vi "WriteOrDestroyStream.vi"(6 "LoopCount":i32, 7 "Clust":T2, 8 "error in (no error)":errorcluster, 9 "Connected":bool, 10 "DataToSend":cluster{"QElmnt":T1, "Data":variant}={"QElmnt"=enum."RTMain_Config", "Data"=variant}, 11 "ref":refnum<k21>) -> (0 "error out":errorcluster, 3 "ref":refnum<k21>)   [LabVIEW 2018]
uses:
  Controls/StreamLoopClust.ctl
  RT/Queue/RTMainQueueElements.ctl
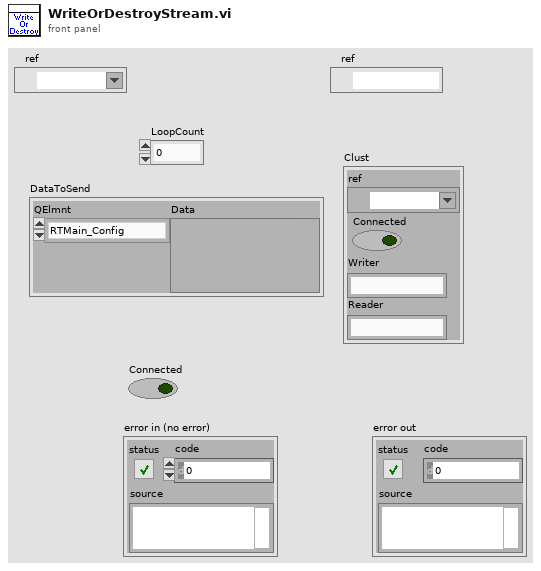
[diagram p1: front panel]
types:
  T1 = typedef "RTMainQueueElements.ctl" = enum16{"RTMain_InitQ", "RTMain_InitSW", "RTMain_InitCtrls", "RTMain_ReInitHW", "RTMain_FromStream", "RTMain_StrtHWLp", "RTMain_UpdtHWClstr", "RTMain_Start", "RTMain_Stop", "RTMain_Error", "RTMain_Config", "RTMain_Exit"}
  T2 = typedef "StreamLoopClust.ctl" = cluster{"ref":refnum<k21>, "Connected":bool, "Writer":string, "Reader":string}
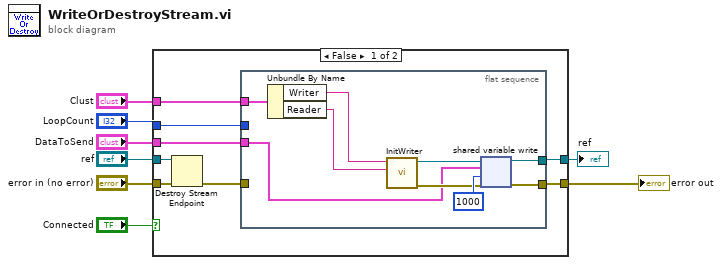
[diagram p0: block diagram]
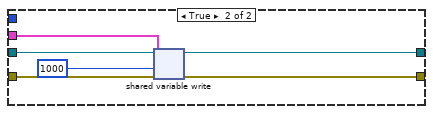
[diagram p2: hidden frame]
diagram:
  n1 = case shown="False" "Connected" {
    tunnel: [w13 w29] -> w1
    tunnel: [w14 w28] -> w6
    tunnel: "DataToSend" -> [w9 w31]
    tunnel: "ref" -> [w15 w26]
    tunnel: "error in (no error)" -> [w16 w30]
    tunnel: "Clust" -> [w12 _]
    tunnel: "LoopCount" -> [w11 _]
    frame False {
      n2 = Destroy Stream Endpoint(8:w16, 11:w15) -> (0:w10:errorcluster)
      n3 = flat-sequence {
        tunnel: [w24] -> w14
        tunnel: [w23] -> w13
        tunnel: w12 -> [w20]
        tunnel: w11 -> [_]
        tunnel: w10 -> [_]
        tunnel: w9 -> [w19]
        frame #0 {
          n4 = Unbundle By Name(w20) -> ("Writer"=w17:string, "Reader"=w18:string)
          n5 = call "InitWriter.vi"("String"=w18, "writer name in"=w17) -> ("error out"=w22:errorcluster, "writer endpoint"=w21:refnum<k21>)  [unwired: 8 in]
          n6 = shared-variable-write(w21, w22, w19, 1000 ("timeout ms (-1)")) -> (w23:refnum<k21>, w24:errorcluster)  [unwired: 1 out]
        }
      }
    }
    frame True {
      n7 = shared-variable-write(w26, w30, w31, 1000 ("timeout ms (-1)")) -> (w29:refnum<k21>, w28:errorcluster)  [unwired: 1 out]
    }
  }
  "error out" <- w6
  "ref" <- w1
